vi "ma_SML RF Spectrum Units Conversion.vi"(6 "spectrum unit in":T2={"units"=enum."Adapt to spectral info", "peak scaling"=enum."rms", "psd?"=FALSE, "impedance(ohm)"=50.0} {"impedance(ohm)" format="%.2f"}, 8 "error in (no error)":errorcluster, 9 "unit conversion settings":T3={"units"=enum."dBV", "peak scaling"=enum."rms", "psd?"=FALSE, "impedance(ohm)"=50.0} {"impedance(ohm)" format="%.2f"}, 10 "spectral info in":T1 {"window" items=["Rectangle"=0, "Hanning"=1, "Hamming"=2, "Blackman-Harris"=3, "Exact Blackman"=4, "Blackman"=5, "Flat Top"=6, "4 Term B-Harris "=7, "7 Term B-Harris"=8, "Low Sidelobe"=9, "Blackman Nuttall"=11, "Triangle"=30, "Bartlett-Hanning"=31, "Bohman"=32, "Parzen"=33, "Welch"=34, "Kaiser"=60, "Dolph-Chebyshev"=61, "Gaussian"=62]}, 11 "power spectrum":T4={"f0"=0.0, "df"=1.0, "spectrum"=[]} {"spectrum" format="%.2f"; "df" format="%.2f"; "f0" format="%.2f"}) -> (0 "error out":errorcluster, 1 "units and label":cluster{"spectrum unit":string, "label":string}={"spectrum unit"="dBV", "label"="dBV rms^2"}, 2 "spectral info out":T1 {"window" items=["Rectangle"=0, "Hanning"=1, "Hamming"=2, "Blackman-Harris"=3, "Exact Blackman"=4, "Blackman"=5, "Flat Top"=6, "4 Term B-Harris "=7, "7 Term B-Harris"=8, "Low Sidelobe"=9, "Blackman Nuttall"=11, "Triangle"=30, "Bartlett-Hanning"=31, "Bohman"=32, "Parzen"=33, "Welch"=34, "Kaiser"=60, "Dolph-Chebyshev"=61, "Gaussian"=62]}, 3 "unit converted spectrum":T4={"f0"=0.0, "df"=1.0, "spectrum"=[]} {"spectrum" format="%.2f"; "df" format="%.2f"; "f0" format="%.2f"})   [LabVIEW 2020, in "NI_MAPro.lvlib"]
uses:
  NI_MAPro.lvlib
  ma_sml_Spectral Info.ctl
  ma_sml_Spectrum Cluster (real).ctl
panel:
  # "RF Spectrum Unit Conversion"
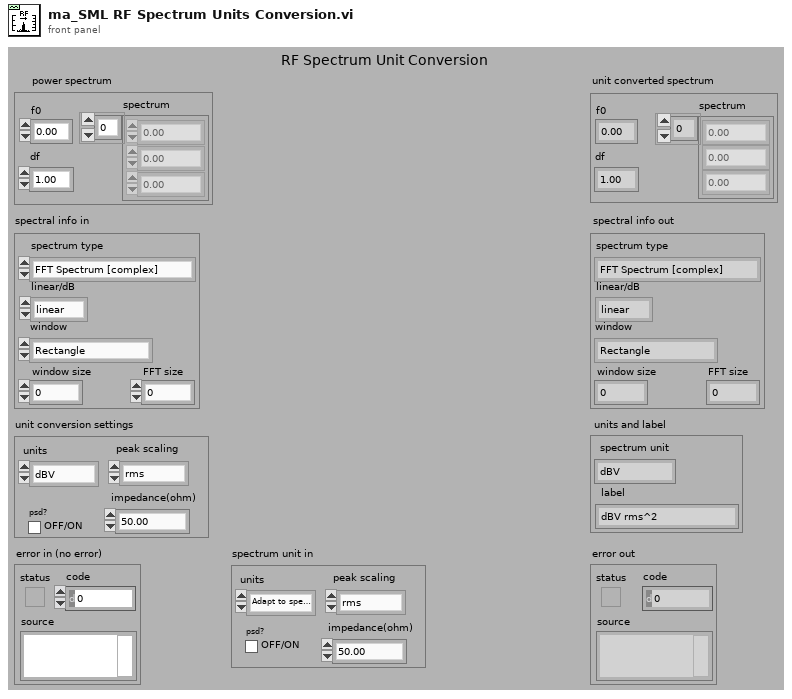
[diagram p1: front panel]
types:
  T1 = typedef "NI_MAPro.lvlib/ma_sml_Spectral Info.ctl" = cluster{"spectrum type":enum16{"FFT Spectrum [complex]", "Amplitude [Magnitude]", "Power [Magnitude^2]", "Cross Spectrum [complex]", "Frequency Response [Complex]"}, "linear/dB":enum16{"linear", "dB"}, "window":u16, "window size":i32, "FFT size":i32}
  T2 = cluster{"units":enum16{"V", "V^2", "W", "dBm", "dBW", "dBV", "dBmV", "dBuV", "Adapt to spectral info"}, "peak scaling":enum16{"rms", "pk"}, "psd?":bool, "impedance(ohm)":dbl}
  T3 = cluster{"units":enum16{"V", "V^2", "W", "dBm", "dBW", "dBV", "dBmV", "dBuV"}, "peak scaling":enum16{"rms", "pk"}, "psd?":bool, "impedance(ohm)":dbl}
  T4 = typedef "NI_MAPro.lvlib/ma_sml_Spectrum Cluster (real).ctl" = cluster{"f0":dbl, "df":dbl, "spectrum":dbl[]}
  T5 = enum16{"FFT Spectrum [complex]", "Amplitude [Magnitude]", "Power [Magnitude^2]", "Cross Spectrum [complex]", "Frequency Response [Complex]"}
  T6 = enum16{"V", "V^2", "W", "dBm", "dBW", "dBV", "dBmV", "dBuV"}
  T7 = enum16{"V", "V^2", "W", "dBm", "dBW", "dBV", "dBmV", "dBuV", "Adapt to spectral info"}
  T8 = enum16{"Linear To Sqr", "Sqr To Linear", "Linear To dB", "dB To Linear", "Sqr To dB", "dB To Sqr", "V^2 To W", "W To V^2", "dBV To dBW", "dBW To dBV", "dB To dBm", "dBm To dB", "dB To dBu", "dBu To dB"}[]
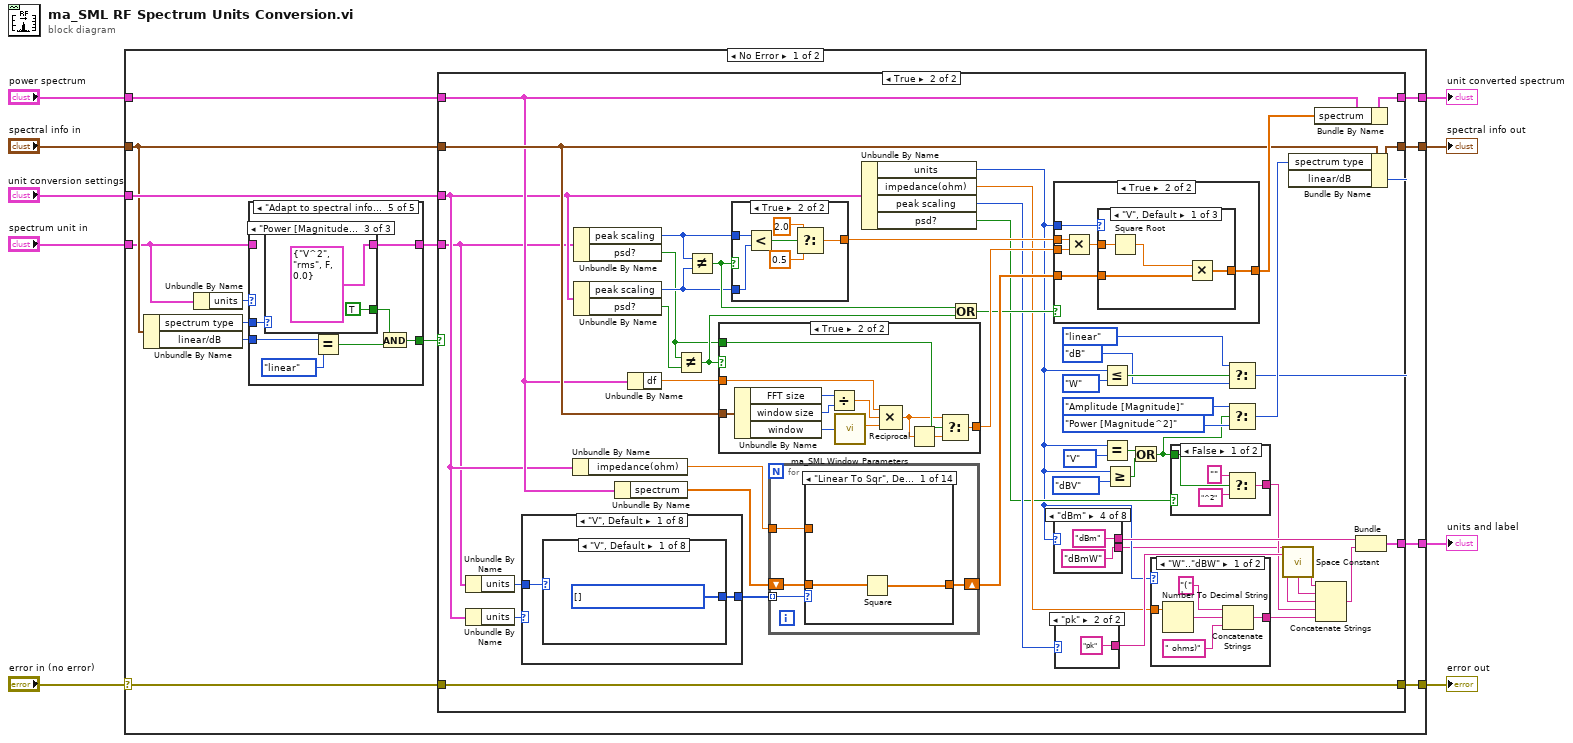
[diagram p0: block diagram]
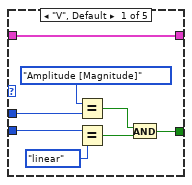
[diagram p2: hidden frame]
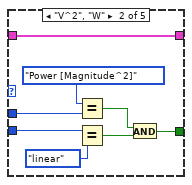
[diagram p3: hidden frame]
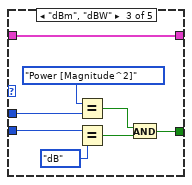
[diagram p4: hidden frame]
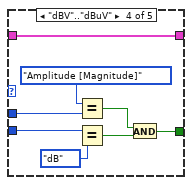
[diagram p5: hidden frame]
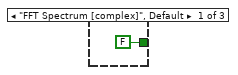
[diagram p6: hidden frame]
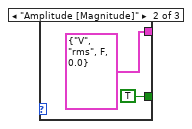
[diagram p7: hidden frame]
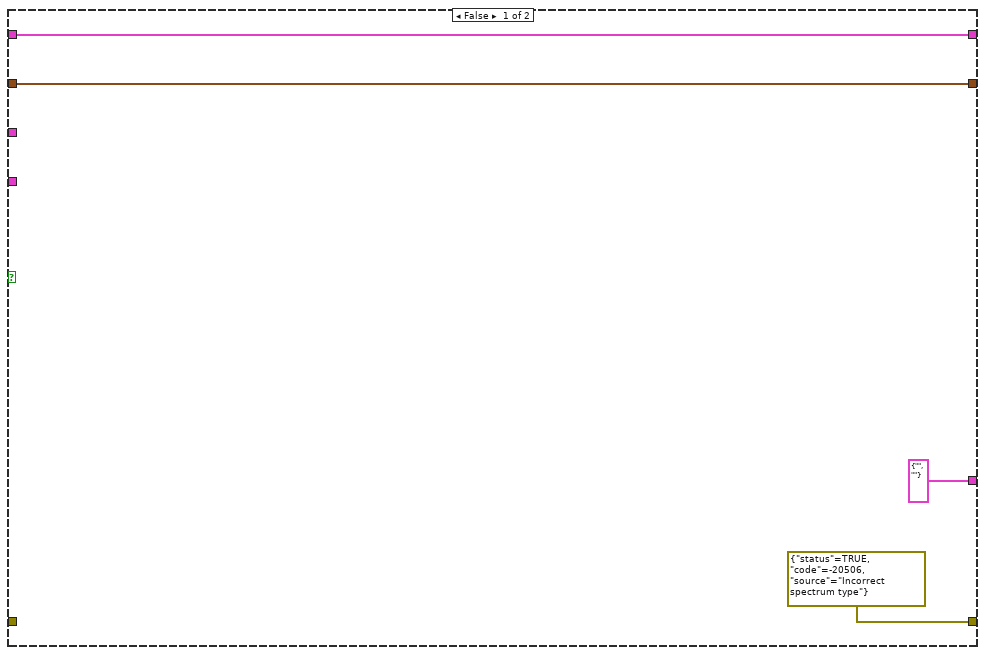
[diagram p8: hidden frame]
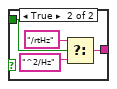
[diagram p9: hidden frame]
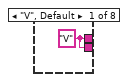
[diagram p10: hidden frame]
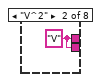
[diagram p11: hidden frame]
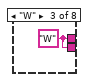
[diagram p12: hidden frame]
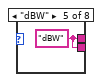
[diagram p13: hidden frame]
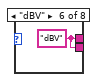
[diagram p14: hidden frame]
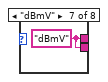
[diagram p15: hidden frame]
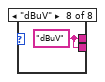
[diagram p16: hidden frame]
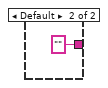
[diagram p17: hidden frame]
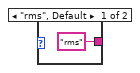
[diagram p18: hidden frame]
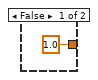
[diagram p19: hidden frame]
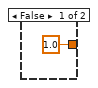
[diagram p20: hidden frame]
diagram:
  n1 = case shown="No Error" "error in (no error)" {
    selector: "error in (no error)" -> [w16 w322]
    tunnel: [w23 w320] -> w9
    tunnel: "power spectrum" -> [w22 w320]
    tunnel: "unit conversion settings" -> [w21 _]
    tunnel: "spectrum unit in" -> [w11 _]
    tunnel: [w20 cluster{string, string} {"", ""}] -> w5
    tunnel: "spectral info in" -> [w18 w321]
    tunnel: [w19 w321] -> w3
    tunnel: [w17 w322] -> w1
    frame No Error {
      n2 = Unbundle By Name(w18) -> ("spectrum type"=w14:T5, "linear/dB"=w13:enum16{"linear", "dB"})
      n3 = Unbundle By Name(w11) -> ("units"=w15:T7)
      n4 = case shown="\"Adapt to spectral info\"" w15 {
        tunnel: w14 -> [w26 w39 w42 w49 w62]
        tunnel: w13 -> [w25 w38 w41 w48 w60]
        tunnel: [w24 w34 w43 w50 w58] -> w12
        tunnel: w11 -> [w31 w35 w40 w55 _]
        tunnel: [w31 w35 w40 w55 w59] -> w10
        frame "V", Default {
          n5 = Equal?(x=T5."Amplitude [Magnitude]", y=w26) -> (x = y?=w27:bool)
          n6 = Equal?(x=w25, y=enum16{"linear", "dB"}."linear") -> (x = y?=w28:bool)
          n7 = And(x=w27, y=w28) -> (x .and. y?=w24:bool)
        }
        frame "V^2", "W" {
          n8 = Equal?(x=T5."Power [Magnitude^2]", y=w39) -> (x = y?=w32:bool)
          n9 = Equal?(x=w38, y=enum16{"linear", "dB"}."linear") -> (x = y?=w33:bool)
          n10 = And(x=w32, y=w33) -> (x .and. y?=w34:bool)
        }
        frame "dBm", "dBW" {
          n11 = Equal?(x=T5."Power [Magnitude^2]", y=w42) -> (x = y?=w44:bool)
          n12 = Equal?(x=w41, y=enum16{"linear", "dB"}."dB") -> (x = y?=w45:bool)
          n13 = And(x=w44, y=w45) -> (x .and. y?=w43:bool)
        }
        frame "dBV".."dBuV" {
          n14 = Equal?(x=T5."Amplitude [Magnitude]", y=w49) -> (x = y?=w51:bool)
          n15 = Equal?(x=w48, y=enum16{"linear", "dB"}."dB") -> (x = y?=w52:bool)
          n16 = And(x=w51, y=w52) -> (x .and. y?=w50:bool)
        }
        frame "Adapt to spectral info" {
          n17 = case shown="\"Power [Magnitude^2]\"" w62 {
            tunnel: [_ T2 {"units"=enum."V", "peak scaling"=enum."rms", "psd?"=FALSE, "impedance(ohm)"=0.0} ("spectrum unit in") T2 {"units"=enum."V^2", "peak scaling"=enum."rms", "psd?"=FALSE, "impedance(ohm)"=0.0} ("spectrum unit in")] -> w59
            tunnel: [FALSE TRUE TRUE] -> w56
            frame "FFT Spectrum [complex]", Default {
            }
            frame "Amplitude [Magnitude]" {
            }
            frame "Power [Magnitude^2]" {
            }
          }
          n18 = Equal?(x=w60, y=enum16{"linear", "dB"}."linear") -> (x = y?=w57:bool)
          n19 = And(x=w56, y=w57) -> (x .and. y?=w58:bool)
        }
      }
      n20 = case shown="True" w12 {
        tunnel: [w70 w120] -> w23
        tunnel: w22 -> [w70 w95]
        tunnel: w21 -> [_ w92]
        tunnel: w10 -> [_ w73]
        tunnel: [cluster{string, string} {"", ""} w101] -> w20
        tunnel: w18 -> [w69 w99]
        tunnel: [w69 w98] -> w19
        tunnel: [errorcluster {"status"=TRUE, "code"=-20506, "source"="Incorrect spectrum type"} ("Output Cluster") w97] -> w17
        tunnel: w16 -> [_ w97]
        frame False {
        }
        frame True {
          n21 = Unbundle By Name(w73) -> ("units"=w118:T7)
          n22 = Unbundle By Name(w92) -> ("units"=w119:T6)
          n23 = case shown="\"V\", Default" w119 {
            tunnel: w118 -> [w186 w195 w205 w215 w225 w235 w245 w255]
            tunnel: [w185 w196 w206 w216 w226 w236 w246 w256] -> w107
            frame "V", Default {
              n24 = case shown="\"V\", Default" w186 {
                tunnel: [w187 w188 w189 w190 w191 w192 w193 w194] -> w185
                frame "V", Default {
                  w187 = T8 [] items=["Linear To Sqr", "Sqr To Linear", "Linear To dB", "dB To Linear", "Sqr To dB", "dB To Sqr", "V^2 To W", "W To V^2", "dBV To dBW", "dBW To dBV", "dB To dBm", "dBm To dB", "dB To dBu", "dBu To dB"]
                }
                frame "V^2" {
                  w188 = T8 [enum."Sqr To Linear"] items=["Linear To Sqr", "Sqr To Linear", "Linear To dB", "dB To Linear", "Sqr To dB", "dB To Sqr", "V^2 To W", "W To V^2", "dBV To dBW", "dBW To dBV", "dB To dBm", "dBm To dB", "dB To dBu", "dBu To dB"]
                }
                frame "W" {
                  w189 = T8 [enum."W To V^2", enum."Sqr To Linear"] items=["Linear To Sqr", "Sqr To Linear", "Linear To dB", "dB To Linear", "Sqr To dB", "dB To Sqr", "V^2 To W", "W To V^2", "dBV To dBW", "dBW To dBV", "dB To dBm", "dBm To dB", "dB To dBu", "dBu To dB"]
                }
                frame "dBm" {
                  w190 = T8 [enum."dBm To dB", enum."dBW To dBV", enum."dB To Linear"] items=["Linear To Sqr", "Sqr To Linear", "Linear To dB", "dB To Linear", "Sqr To dB", "dB To Sqr", "V^2 To W", "W To V^2", "dBV To dBW", "dBW To dBV", "dB To dBm", "dBm To dB", "dB To dBu", "dBu To dB"]
                }
                frame "dBW" {
                  w191 = T8 [enum."dBW To dBV", enum."dB To Linear"] items=["Linear To Sqr", "Sqr To Linear", "Linear To dB", "dB To Linear", "Sqr To dB", "dB To Sqr", "V^2 To W", "W To V^2", "dBV To dBW", "dBW To dBV", "dB To dBm", "dBm To dB", "dB To dBu", "dBu To dB"]
                }
                frame "dBV" {
                  w192 = T8 [enum."dB To Linear"] items=["Linear To Sqr", "Sqr To Linear", "Linear To dB", "dB To Linear", "Sqr To dB", "dB To Sqr", "V^2 To W", "W To V^2", "dBV To dBW", "dBW To dBV", "dB To dBm", "dBm To dB", "dB To dBu", "dBu To dB"]
                }
                frame "dBmV" {
                  w193 = T8 [enum."dBu To dB", enum."dB To Linear"] items=["Linear To Sqr", "Sqr To Linear", "Linear To dB", "dB To Linear", "Sqr To dB", "dB To Sqr", "V^2 To W", "W To V^2", "dBV To dBW", "dBW To dBV", "dB To dBm", "dBm To dB", "dB To dBu", "dBu To dB"]
                }
                frame "dBuV" {
                  w194 = T8 [enum."dBu To dB", enum."dBu To dB", enum."dB To Linear"] items=["Linear To Sqr", "Sqr To Linear", "Linear To dB", "dB To Linear", "Sqr To dB", "dB To Sqr", "V^2 To W", "W To V^2", "dBV To dBW", "dBW To dBV", "dB To dBm", "dBm To dB", "dB To dBu", "dBu To dB"]
                }
              }
            }
            frame "V^2" {
              n25 = case shown="\"V\", Default" w195 {
                tunnel: [w197 w198 w199 w200 w201 w202 w203 w204] -> w196
                frame "V", Default {
                  w197 = T8 [enum."Linear To Sqr"] items=["Linear To Sqr", "Sqr To Linear", "Linear To dB", "dB To Linear", "Sqr To dB", "dB To Sqr", "V^2 To W", "W To V^2", "dBV To dBW", "dBW To dBV", "dB To dBm", "dBm To dB", "dB To dBu", "dBu To dB"]
                }
                frame "V^2" {
                  w198 = T8 [] items=["Linear To Sqr", "Sqr To Linear", "Linear To dB", "dB To Linear", "Sqr To dB", "dB To Sqr", "V^2 To W", "W To V^2", "dBV To dBW", "dBW To dBV", "dB To dBm", "dBm To dB", "dB To dBu", "dBu To dB"]
                }
                frame "W" {
                  w199 = T8 [enum."W To V^2"] items=["Linear To Sqr", "Sqr To Linear", "Linear To dB", "dB To Linear", "Sqr To dB", "dB To Sqr", "V^2 To W", "W To V^2", "dBV To dBW", "dBW To dBV", "dB To dBm", "dBm To dB", "dB To dBu", "dBu To dB"]
                }
                frame "dBm" {
                  w200 = T8 [enum."dBm To dB", enum."dBW To dBV", enum."dB To Sqr"] items=["Linear To Sqr", "Sqr To Linear", "Linear To dB", "dB To Linear", "Sqr To dB", "dB To Sqr", "V^2 To W", "W To V^2", "dBV To dBW", "dBW To dBV", "dB To dBm", "dBm To dB", "dB To dBu", "dBu To dB"]
                }
                frame "dBW" {
                  w201 = T8 [enum."dBW To dBV", enum."dB To Sqr"] items=["Linear To Sqr", "Sqr To Linear", "Linear To dB", "dB To Linear", "Sqr To dB", "dB To Sqr", "V^2 To W", "W To V^2", "dBV To dBW", "dBW To dBV", "dB To dBm", "dBm To dB", "dB To dBu", "dBu To dB"]
                }
                frame "dBV" {
                  w202 = T8 [enum."dB To Sqr"] items=["Linear To Sqr", "Sqr To Linear", "Linear To dB", "dB To Linear", "Sqr To dB", "dB To Sqr", "V^2 To W", "W To V^2", "dBV To dBW", "dBW To dBV", "dB To dBm", "dBm To dB", "dB To dBu", "dBu To dB"]
                }
                frame "dBmV" {
                  w203 = T8 [enum."dBu To dB", enum."dB To Sqr"] items=["Linear To Sqr", "Sqr To Linear", "Linear To dB", "dB To Linear", "Sqr To dB", "dB To Sqr", "V^2 To W", "W To V^2", "dBV To dBW", "dBW To dBV", "dB To dBm", "dBm To dB", "dB To dBu", "dBu To dB"]
                }
                frame "dBuV" {
                  w204 = T8 [enum."dBu To dB", enum."dBu To dB", enum."dB To Sqr"] items=["Linear To Sqr", "Sqr To Linear", "Linear To dB", "dB To Linear", "Sqr To dB", "dB To Sqr", "V^2 To W", "W To V^2", "dBV To dBW", "dBW To dBV", "dB To dBm", "dBm To dB", "dB To dBu", "dBu To dB"]
                }
              }
            }
            frame "W" {
              n26 = case shown="\"V\", Default" w205 {
                tunnel: [w207 w208 w209 w210 w211 w212 w213 w214] -> w206
                frame "V", Default {
                  w207 = T8 [enum."Linear To Sqr", enum."V^2 To W"] items=["Linear To Sqr", "Sqr To Linear", "Linear To dB", "dB To Linear", "Sqr To dB", "dB To Sqr", "V^2 To W", "W To V^2", "dBV To dBW", "dBW To dBV", "dB To dBm", "dBm To dB", "dB To dBu", "dBu To dB"]
                }
                frame "V^2" {
                  w208 = T8 [enum."V^2 To W"] items=["Linear To Sqr", "Sqr To Linear", "Linear To dB", "dB To Linear", "Sqr To dB", "dB To Sqr", "V^2 To W", "W To V^2", "dBV To dBW", "dBW To dBV", "dB To dBm", "dBm To dB", "dB To dBu", "dBu To dB"]
                }
                frame "W" {
                  w209 = T8 [] items=["Linear To Sqr", "Sqr To Linear", "Linear To dB", "dB To Linear", "Sqr To dB", "dB To Sqr", "V^2 To W", "W To V^2", "dBV To dBW", "dBW To dBV", "dB To dBm", "dBm To dB", "dB To dBu", "dBu To dB"]
                }
                frame "dBm" {
                  w210 = T8 [enum."dBm To dB", enum."dB To Sqr"] items=["Linear To Sqr", "Sqr To Linear", "Linear To dB", "dB To Linear", "Sqr To dB", "dB To Sqr", "V^2 To W", "W To V^2", "dBV To dBW", "dBW To dBV", "dB To dBm", "dBm To dB", "dB To dBu", "dBu To dB"]
                }
                frame "dBW" {
                  w211 = T8 [enum."dB To Sqr"] items=["Linear To Sqr", "Sqr To Linear", "Linear To dB", "dB To Linear", "Sqr To dB", "dB To Sqr", "V^2 To W", "W To V^2", "dBV To dBW", "dBW To dBV", "dB To dBm", "dBm To dB", "dB To dBu", "dBu To dB"]
                }
                frame "dBV" {
                  w212 = T8 [enum."dBV To dBW", enum."dB To Sqr"] items=["Linear To Sqr", "Sqr To Linear", "Linear To dB", "dB To Linear", "Sqr To dB", "dB To Sqr", "V^2 To W", "W To V^2", "dBV To dBW", "dBW To dBV", "dB To dBm", "dBm To dB", "dB To dBu", "dBu To dB"]
                }
                frame "dBmV" {
                  w213 = T8 [enum."dBu To dB", enum."dBV To dBW", enum."dB To Sqr"] items=["Linear To Sqr", "Sqr To Linear", "Linear To dB", "dB To Linear", "Sqr To dB", "dB To Sqr", "V^2 To W", "W To V^2", "dBV To dBW", "dBW To dBV", "dB To dBm", "dBm To dB", "dB To dBu", "dBu To dB"]
                }
                frame "dBuV" {
                  w214 = T8 [enum."dBu To dB", enum."dBu To dB", enum."dBV To dBW", enum."dB To Sqr"] items=["Linear To Sqr", "Sqr To Linear", "Linear To dB", "dB To Linear", "Sqr To dB", "dB To Sqr", "V^2 To W", "W To V^2", "dBV To dBW", "dBW To dBV", "dB To dBm", "dBm To dB", "dB To dBu", "dBu To dB"]
                }
              }
            }
            frame "dBm" {
              n27 = case shown="\"V\", Default" w215 {
                tunnel: [w217 w218 w219 w220 w221 w222 w223 w224] -> w216
                frame "V", Default {
                  w217 = T8 [enum."Linear To dB", enum."dBV To dBW", enum."dB To dBm"] items=["Linear To Sqr", "Sqr To Linear", "Linear To dB", "dB To Linear", "Sqr To dB", "dB To Sqr", "V^2 To W", "W To V^2", "dBV To dBW", "dBW To dBV", "dB To dBm", "dBm To dB", "dB To dBu", "dBu To dB"]
                }
                frame "V^2" {
                  w218 = T8 [enum."Sqr To dB", enum."dBV To dBW", enum."dB To dBm"] items=["Linear To Sqr", "Sqr To Linear", "Linear To dB", "dB To Linear", "Sqr To dB", "dB To Sqr", "V^2 To W", "W To V^2", "dBV To dBW", "dBW To dBV", "dB To dBm", "dBm To dB", "dB To dBu", "dBu To dB"]
                }
                frame "W" {
                  w219 = T8 [enum."Sqr To dB", enum."dB To dBm"] items=["Linear To Sqr", "Sqr To Linear", "Linear To dB", "dB To Linear", "Sqr To dB", "dB To Sqr", "V^2 To W", "W To V^2", "dBV To dBW", "dBW To dBV", "dB To dBm", "dBm To dB", "dB To dBu", "dBu To dB"]
                }
                frame "dBm" {
                  w220 = T8 [] items=["Linear To Sqr", "Sqr To Linear", "Linear To dB", "dB To Linear", "Sqr To dB", "dB To Sqr", "V^2 To W", "W To V^2", "dBV To dBW", "dBW To dBV", "dB To dBm", "dBm To dB", "dB To dBu", "dBu To dB"]
                }
                frame "dBW" {
                  w221 = T8 [enum."dB To dBm"] items=["Linear To Sqr", "Sqr To Linear", "Linear To dB", "dB To Linear", "Sqr To dB", "dB To Sqr", "V^2 To W", "W To V^2", "dBV To dBW", "dBW To dBV", "dB To dBm", "dBm To dB", "dB To dBu", "dBu To dB"]
                }
                frame "dBV" {
                  w222 = T8 [enum."dBV To dBW", enum."dB To dBm"] items=["Linear To Sqr", "Sqr To Linear", "Linear To dB", "dB To Linear", "Sqr To dB", "dB To Sqr", "V^2 To W", "W To V^2", "dBV To dBW", "dBW To dBV", "dB To dBm", "dBm To dB", "dB To dBu", "dBu To dB"]
                }
                frame "dBmV" {
                  w223 = T8 [enum."dBV To dBW", enum."dBm To dB"] items=["Linear To Sqr", "Sqr To Linear", "Linear To dB", "dB To Linear", "Sqr To dB", "dB To Sqr", "V^2 To W", "W To V^2", "dBV To dBW", "dBW To dBV", "dB To dBm", "dBm To dB", "dB To dBu", "dBu To dB"]
                }
                frame "dBuV" {
                  w224 = T8 [enum."dBV To dBW", enum."dBm To dB", enum."dBu To dB"] items=["Linear To Sqr", "Sqr To Linear", "Linear To dB", "dB To Linear", "Sqr To dB", "dB To Sqr", "V^2 To W", "W To V^2", "dBV To dBW", "dBW To dBV", "dB To dBm", "dBm To dB", "dB To dBu", "dBu To dB"]
                }
              }
            }
            frame "dBW" {
              n28 = case shown="\"V\", Default" w225 {
                tunnel: [w227 w228 w229 w230 w231 w232 w233 w234] -> w226
                frame "V", Default {
                  w227 = T8 [enum."Linear To dB", enum."dBV To dBW"] items=["Linear To Sqr", "Sqr To Linear", "Linear To dB", "dB To Linear", "Sqr To dB", "dB To Sqr", "V^2 To W", "W To V^2", "dBV To dBW", "dBW To dBV", "dB To dBm", "dBm To dB", "dB To dBu", "dBu To dB"]
                }
                frame "V^2" {
                  w228 = T8 [enum."Sqr To dB", enum."dBV To dBW"] items=["Linear To Sqr", "Sqr To Linear", "Linear To dB", "dB To Linear", "Sqr To dB", "dB To Sqr", "V^2 To W", "W To V^2", "dBV To dBW", "dBW To dBV", "dB To dBm", "dBm To dB", "dB To dBu", "dBu To dB"]
                }
                frame "W" {
                  w229 = T8 [enum."Sqr To dB"] items=["Linear To Sqr", "Sqr To Linear", "Linear To dB", "dB To Linear", "Sqr To dB", "dB To Sqr", "V^2 To W", "W To V^2", "dBV To dBW", "dBW To dBV", "dB To dBm", "dBm To dB", "dB To dBu", "dBu To dB"]
                }
                frame "dBm" {
                  w230 = T8 [enum."dBm To dB"] items=["Linear To Sqr", "Sqr To Linear", "Linear To dB", "dB To Linear", "Sqr To dB", "dB To Sqr", "V^2 To W", "W To V^2", "dBV To dBW", "dBW To dBV", "dB To dBm", "dBm To dB", "dB To dBu", "dBu To dB"]
                }
                frame "dBW" {
                  w231 = T8 [] items=["Linear To Sqr", "Sqr To Linear", "Linear To dB", "dB To Linear", "Sqr To dB", "dB To Sqr", "V^2 To W", "W To V^2", "dBV To dBW", "dBW To dBV", "dB To dBm", "dBm To dB", "dB To dBu", "dBu To dB"]
                }
                frame "dBV" {
                  w232 = T8 [enum."dBV To dBW"] items=["Linear To Sqr", "Sqr To Linear", "Linear To dB", "dB To Linear", "Sqr To dB", "dB To Sqr", "V^2 To W", "W To V^2", "dBV To dBW", "dBW To dBV", "dB To dBm", "dBm To dB", "dB To dBu", "dBu To dB"]
                }
                frame "dBmV" {
                  w233 = T8 [enum."dBV To dBW", enum."dBu To dB"] items=["Linear To Sqr", "Sqr To Linear", "Linear To dB", "dB To Linear", "Sqr To dB", "dB To Sqr", "V^2 To W", "W To V^2", "dBV To dBW", "dBW To dBV", "dB To dBm", "dBm To dB", "dB To dBu", "dBu To dB"]
                }
                frame "dBuV" {
                  w234 = T8 [enum."dBV To dBW", enum."dBu To dB", enum."dBu To dB"] items=["Linear To Sqr", "Sqr To Linear", "Linear To dB", "dB To Linear", "Sqr To dB", "dB To Sqr", "V^2 To W", "W To V^2", "dBV To dBW", "dBW To dBV", "dB To dBm", "dBm To dB", "dB To dBu", "dBu To dB"]
                }
              }
            }
            frame "dBV" {
              n29 = case shown="\"V\", Default" w235 {
                tunnel: [w237 w238 w239 w240 w241 w242 w243 w244] -> w236
                frame "V", Default {
                  w237 = T8 [enum."Linear To dB"] items=["Linear To Sqr", "Sqr To Linear", "Linear To dB", "dB To Linear", "Sqr To dB", "dB To Sqr", "V^2 To W", "W To V^2", "dBV To dBW", "dBW To dBV", "dB To dBm", "dBm To dB", "dB To dBu", "dBu To dB"]
                }
                frame "V^2" {
                  w238 = T8 [enum."Sqr To dB"] items=["Linear To Sqr", "Sqr To Linear", "Linear To dB", "dB To Linear", "Sqr To dB", "dB To Sqr", "V^2 To W", "W To V^2", "dBV To dBW", "dBW To dBV", "dB To dBm", "dBm To dB", "dB To dBu", "dBu To dB"]
                }
                frame "W" {
                  w239 = T8 [enum."Sqr To dB", enum."dBW To dBV"] items=["Linear To Sqr", "Sqr To Linear", "Linear To dB", "dB To Linear", "Sqr To dB", "dB To Sqr", "V^2 To W", "W To V^2", "dBV To dBW", "dBW To dBV", "dB To dBm", "dBm To dB", "dB To dBu", "dBu To dB"]
                }
                frame "dBm" {
                  w240 = T8 [enum."dBW To dBV", enum."dBm To dB"] items=["Linear To Sqr", "Sqr To Linear", "Linear To dB", "dB To Linear", "Sqr To dB", "dB To Sqr", "V^2 To W", "W To V^2", "dBV To dBW", "dBW To dBV", "dB To dBm", "dBm To dB", "dB To dBu", "dBu To dB"]
                }
                frame "dBW" {
                  w241 = T8 [enum."dBW To dBV"] items=["Linear To Sqr", "Sqr To Linear", "Linear To dB", "dB To Linear", "Sqr To dB", "dB To Sqr", "V^2 To W", "W To V^2", "dBV To dBW", "dBW To dBV", "dB To dBm", "dBm To dB", "dB To dBu", "dBu To dB"]
                }
                frame "dBV" {
                  w242 = T8 [] items=["Linear To Sqr", "Sqr To Linear", "Linear To dB", "dB To Linear", "Sqr To dB", "dB To Sqr", "V^2 To W", "W To V^2", "dBV To dBW", "dBW To dBV", "dB To dBm", "dBm To dB", "dB To dBu", "dBu To dB"]
                }
                frame "dBmV" {
                  w243 = T8 [enum."dBu To dB"] items=["Linear To Sqr", "Sqr To Linear", "Linear To dB", "dB To Linear", "Sqr To dB", "dB To Sqr", "V^2 To W", "W To V^2", "dBV To dBW", "dBW To dBV", "dB To dBm", "dBm To dB", "dB To dBu", "dBu To dB"]
                }
                frame "dBuV" {
                  w244 = T8 [enum."dBu To dB", enum."dBu To dB"] items=["Linear To Sqr", "Sqr To Linear", "Linear To dB", "dB To Linear", "Sqr To dB", "dB To Sqr", "V^2 To W", "W To V^2", "dBV To dBW", "dBW To dBV", "dB To dBm", "dBm To dB", "dB To dBu", "dBu To dB"]
                }
              }
            }
            frame "dBmV" {
              n30 = case shown="\"V\", Default" w245 {
                tunnel: [w247 w248 w249 w250 w251 w252 w253 w254] -> w246
                frame "V", Default {
                  w247 = T8 [enum."Linear To dB", enum."dB To dBu"] items=["Linear To Sqr", "Sqr To Linear", "Linear To dB", "dB To Linear", "Sqr To dB", "dB To Sqr", "V^2 To W", "W To V^2", "dBV To dBW", "dBW To dBV", "dB To dBm", "dBm To dB", "dB To dBu", "dBu To dB"]
                }
                frame "V^2" {
                  w248 = T8 [enum."Sqr To dB", enum."dB To dBu"] items=["Linear To Sqr", "Sqr To Linear", "Linear To dB", "dB To Linear", "Sqr To dB", "dB To Sqr", "V^2 To W", "W To V^2", "dBV To dBW", "dBW To dBV", "dB To dBm", "dBm To dB", "dB To dBu", "dBu To dB"]
                }
                frame "W" {
                  w249 = T8 [enum."Sqr To dB", enum."dBW To dBV", enum."dB To dBu"] items=["Linear To Sqr", "Sqr To Linear", "Linear To dB", "dB To Linear", "Sqr To dB", "dB To Sqr", "V^2 To W", "W To V^2", "dBV To dBW", "dBW To dBV", "dB To dBm", "dBm To dB", "dB To dBu", "dBu To dB"]
                }
                frame "dBm" {
                  w250 = T8 [enum."dBW To dBV", enum."dB To dBm"] items=["Linear To Sqr", "Sqr To Linear", "Linear To dB", "dB To Linear", "Sqr To dB", "dB To Sqr", "V^2 To W", "W To V^2", "dBV To dBW", "dBW To dBV", "dB To dBm", "dBm To dB", "dB To dBu", "dBu To dB"]
                }
                frame "dBW" {
                  w251 = T8 [enum."dBW To dBV", enum."dB To dBu"] items=["Linear To Sqr", "Sqr To Linear", "Linear To dB", "dB To Linear", "Sqr To dB", "dB To Sqr", "V^2 To W", "W To V^2", "dBV To dBW", "dBW To dBV", "dB To dBm", "dBm To dB", "dB To dBu", "dBu To dB"]
                }
                frame "dBV" {
                  w252 = T8 [enum."dB To dBu"] items=["Linear To Sqr", "Sqr To Linear", "Linear To dB", "dB To Linear", "Sqr To dB", "dB To Sqr", "V^2 To W", "W To V^2", "dBV To dBW", "dBW To dBV", "dB To dBm", "dBm To dB", "dB To dBu", "dBu To dB"]
                }
                frame "dBmV" {
                  w253 = T8 [] items=["Linear To Sqr", "Sqr To Linear", "Linear To dB", "dB To Linear", "Sqr To dB", "dB To Sqr", "V^2 To W", "W To V^2", "dBV To dBW", "dBW To dBV", "dB To dBm", "dBm To dB", "dB To dBu", "dBu To dB"]
                }
                frame "dBuV" {
                  w254 = T8 [enum."dBu To dB"] items=["Linear To Sqr", "Sqr To Linear", "Linear To dB", "dB To Linear", "Sqr To dB", "dB To Sqr", "V^2 To W", "W To V^2", "dBV To dBW", "dBW To dBV", "dB To dBm", "dBm To dB", "dB To dBu", "dBu To dB"]
                }
              }
            }
            frame "dBuV" {
              n31 = case shown="\"V\", Default" w255 {
                tunnel: [w257 w258 w259 w260 w261 w262 w263 w264] -> w256
                frame "V", Default {
                  w257 = T8 [enum."Linear To dB", enum."dB To dBu", enum."dB To dBu"] items=["Linear To Sqr", "Sqr To Linear", "Linear To dB", "dB To Linear", "Sqr To dB", "dB To Sqr", "V^2 To W", "W To V^2", "dBV To dBW", "dBW To dBV", "dB To dBm", "dBm To dB", "dB To dBu", "dBu To dB"]
                }
                frame "V^2" {
                  w258 = T8 [enum."Sqr To dB", enum."dB To dBu", enum."dB To dBu"] items=["Linear To Sqr", "Sqr To Linear", "Linear To dB", "dB To Linear", "Sqr To dB", "dB To Sqr", "V^2 To W", "W To V^2", "dBV To dBW", "dBW To dBV", "dB To dBm", "dBm To dB", "dB To dBu", "dBu To dB"]
                }
                frame "W" {
                  w259 = T8 [enum."Sqr To dB", enum."dBW To dBV", enum."dB To dBu", enum."dB To dBu"] items=["Linear To Sqr", "Sqr To Linear", "Linear To dB", "dB To Linear", "Sqr To dB", "dB To Sqr", "V^2 To W", "W To V^2", "dBV To dBW", "dBW To dBV", "dB To dBm", "dBm To dB", "dB To dBu", "dBu To dB"]
                }
                frame "dBm" {
                  w260 = T8 [enum."dBW To dBV", enum."dB To dBm", enum."dB To dBu"] items=["Linear To Sqr", "Sqr To Linear", "Linear To dB", "dB To Linear", "Sqr To dB", "dB To Sqr", "V^2 To W", "W To V^2", "dBV To dBW", "dBW To dBV", "dB To dBm", "dBm To dB", "dB To dBu", "dBu To dB"]
                }
                frame "dBW" {
                  w261 = T8 [enum."dBW To dBV", enum."dB To dBu", enum."dB To dBu"] items=["Linear To Sqr", "Sqr To Linear", "Linear To dB", "dB To Linear", "Sqr To dB", "dB To Sqr", "V^2 To W", "W To V^2", "dBV To dBW", "dBW To dBV", "dB To dBm", "dBm To dB", "dB To dBu", "dBu To dB"]
                }
                frame "dBV" {
                  w262 = T8 [enum."dB To dBu", enum."dB To dBu"] items=["Linear To Sqr", "Sqr To Linear", "Linear To dB", "dB To Linear", "Sqr To dB", "dB To Sqr", "V^2 To W", "W To V^2", "dBV To dBW", "dBW To dBV", "dB To dBm", "dBm To dB", "dB To dBu", "dBu To dB"]
                }
                frame "dBmV" {
                  w263 = T8 [enum."dB To dBu"] items=["Linear To Sqr", "Sqr To Linear", "Linear To dB", "dB To Linear", "Sqr To dB", "dB To Sqr", "V^2 To W", "W To V^2", "dBV To dBW", "dBW To dBV", "dB To dBm", "dBm To dB", "dB To dBu", "dBu To dB"]
                }
                frame "dBuV" {
                  w264 = T8 [] items=["Linear To Sqr", "Sqr To Linear", "Linear To dB", "dB To Linear", "Sqr To dB", "dB To Sqr", "V^2 To W", "W To V^2", "dBV To dBW", "dBW To dBV", "dB To dBm", "dBm To dB", "dB To dBu", "dBu To dB"]
                }
              }
            }
          }
          n32 = Unbundle By Name(w92) -> ("impedance(ohm)"=w93:dbl)
          n33 = Unbundle By Name(w73) -> ("peak scaling"=w111:enum16{"rms", "pk"}, "psd?"=w96:bool)
          n34 = Unbundle By Name(w92) -> ("peak scaling"=w110:enum16{"rms", "pk"}, "psd?"=w109:bool)
          n35 = Unbundle By Name(w95) -> ("spectrum"=w108:dbl[])
          n36 = Unbundle By Name(w95) -> ("df"=w94:dbl)
          n37 = Not Equal?(x=w96, y=w109) -> (x != y?=w115:bool)
          n38 = Not Equal?(x=w111, y=w110) -> (x != y?=w116:bool)
          n39 = case shown="True" w115 {
            tunnel: w96 -> [_ w151]
            tunnel: w99 -> [_ w157]
            tunnel: [1.0 w150] -> w113
            tunnel: w94 -> [_ w149]
            frame False {
            }
            frame True {
              n40 = Unbundle By Name(w157) -> ("FFT size"=w156:i32, "window size"=w155:i32, "window"=w154:u16)
              n41 = Divide(x=w156, y=w155) -> (x/y=w153:dbl)
              n42 = call "ma_SML Window Parameters.vi"("window"=w154) -> ("ENBW"=w152:dbl)  [unwired: 3 out]
              n43 = Compound Arithmetic op=MULTIPLY(w149, w153, w152) -> (w147:dbl)
              n44 = Reciprocal(x=w147) -> (1/x=w148:dbl)
              n45 = Select(t=w147, s=w151, f=w148) -> (s? t:f=w150:dbl)
            }
          }
          n46 = case shown="True" w116 {
            tunnel: w111 -> [_ w161]
            tunnel: w110 -> [_ w160]
            tunnel: [1.0 w159] -> w114
            frame False {
            }
            frame True {
              n47 = Less?(x=w161, y=w160) -> (x < y?=w163:bool)
              n48 = Select(t=2.0, s=w163, f=0.5) -> (s? t:f=w159:dbl)
            }
          }
          n49 = for {
            shift-right: [w267] -> w117
            shift-left: w108 -> [w268]
            tunnel: w93 -> [w266]
            tunnel: w107 -> [w265] mode=indexing
            n50 = case shown="\"Linear To Sqr\", Default" w265 {
              tunnel: w268 -> [w270 w272 w276 w278 w284 w287 w291 w293 w296 w304 w308 w312 w315 w318]
              tunnel: [w269 w271 w275 w277 w283 w286 w290 w294 w299 w302 w309 w311 w314 w316] -> w267
              tunnel: w266 -> [_ _ _ _ _ _ w289 w292 w295 w301 _ _ _ _]
              frame "Linear To Sqr", Default {
                n51 = Square(x=w270) -> (x^2=w269:dbl[])
              }
              frame "Sqr To Linear" {
                n52 = Square Root(x=w272) -> (sqrt(x)=w271:dbl[])
              }
              frame "Linear To dB" {
                n53 = Logarithm Base 10(1:w276) -> (0:w274:dbl[])
                n54 = Multiply(x=20.0, y=w274) -> (x*y=w275:dbl[])
              }
              frame "dB To Linear" {
                n55 = Divide(x=w278, y=20.0) -> (x/y=w279:dbl[])
                n56 = Power Of 10(x=w279) -> (10^x=w277:dbl[])
              }
              frame "Sqr To dB" {
                n57 = Logarithm Base 10(1:w284) -> (0:w282:dbl[])
                n58 = Multiply(x=10.0, y=w282) -> (x*y=w283:dbl[])
              }
              frame "dB To Sqr" {
                n59 = Divide(x=w287, y=10.0) -> (x/y=w285:dbl[])
                n60 = Power Of 10(x=w285) -> (10^x=w286:dbl[])
              }
              frame "V^2 To W" {
                n61 = Divide(x=w291, y=w289) -> (x/y=w290:dbl[])
              }
              frame "W To V^2" {
                n62 = Multiply(x=w292, y=w293) -> (x*y=w294:dbl[])
              }
              frame "dBV To dBW" {
                n63 = Logarithm Base 10(1:w295) -> (0:w298:dbl)
                n64 = Multiply(x=10.0 ("y"), y=w298) -> (x*y=w300:dbl)
                n65 = Subtract(x=w296, y=w300) -> (x-y=w299:dbl[])
              }
              frame "dBW To dBV" {
                n66 = Logarithm Base 10(1:w301) -> (0:w306:dbl)
                n67 = Multiply(x=10.0 ("y"), y=w306) -> (x*y=w303:dbl)
                n68 = Add(x=w303, y=w304) -> (x+y=w302:dbl[])
              }
              frame "dB To dBm" {
                n69 = Add(x=w308, y=30.0) -> (x+y=w309:dbl[])
              }
              frame "dBm To dB" {
                n70 = Subtract(x=w312, y=30.0) -> (x-y=w311:dbl[])
              }
              frame "dB To dBu" {
                n71 = Add(x=w315, y=60.0) -> (x+y=w314:dbl[])
              }
              frame "dBu To dB" {
                n72 = Subtract(x=w318, y=60.0) -> (x-y=w316:dbl[])
              }
            }
          }
          n73 = Unbundle By Name(w92) -> ("units"=w76:T6, "impedance(ohm)"=w105:dbl, "peak scaling"=w90:enum16{"rms", "pk"}, "psd?"=w80:bool)
          n74 = Or(x=w116, y=w115) -> (x .or. y?=w112:bool)
          n75 = case shown="True" w112 {
            tunnel: w117 -> [w165 w171]
            tunnel: [w165 w170] -> w100
            tunnel: w114 -> [_ w167]
            tunnel: w113 -> [_ w169]
            tunnel: w76 -> [_ w166]
            frame False {
            }
            frame True {
              n76 = Multiply(x=w167, y=w169) -> (x*y=w168:dbl)
              n77 = case shown="\"V\", Default" w166 {
                tunnel: w168 -> [w175 w177 w181]
                tunnel: w171 -> [w173 w178 w184]
                tunnel: [w172 w176 w183] -> w170
                frame "V", Default {
                  n78 = Square Root(x=w175) -> (sqrt(x)=w174:dbl)
                  n79 = Multiply(x=w174, y=w173) -> (x*y=w172:dbl[])
                }
                frame "V^2", "W" {
                  n80 = Multiply(x=w177, y=w178) -> (x*y=w176:dbl[])
                }
                frame "dBm".."dBuV" {
                  n81 = Logarithm Base 10(1:w181) -> (0:w182:dbl)
                  n82 = Multiply(x=w182, y=10.0) -> (x*y=w180:dbl)
                  n83 = Add(x=w180, y=w184) -> (x+y=w183:dbl[])
                }
              }
            }
          }
          n84 = case shown="\"dBm\"" w76 {
            tunnel: [w129 w130 w131 "dBm" w134 w135 w136 w137] -> w103
            tunnel: [w129 w130 w131 "dBmW" w134 w135 w136 w137] -> w72
            frame "V", Default {
              w129 = "V"
            }
            frame "V^2" {
              w130 = "V"
            }
            frame "W" {
              w131 = "W"
            }
            frame "dBm" {
            }
            frame "dBW" {
              w134 = "dBW"
            }
            frame "dBV" {
              w135 = "dBV"
            }
            frame "dBmV" {
              w136 = "dBmV"
            }
            frame "dBuV" {
              w137 = "dBuV"
            }
          }
          n85 = case shown="\"pk\"" w90 {
            tunnel: ["rms" "pk"] -> w106
            frame "rms", Default {
            }
            frame "pk" {
            }
          }
          n86 = Less Or Equal?(x=w76, y=T6."W") -> (x <= y?=w85:bool)
          n87 = Equal?(x=w76, y=T6."V") -> (x = y?=w75:bool)
          n88 = Greater Or Equal?(x=w76, y=T6."dBV") -> (x >= y?=w77:bool)
          n89 = Or(x=w75, y=w77) -> (x .or. y?=w74:bool)
          n90 = case shown="\"W\"..\"dBW\"" w76 {
            tunnel: w105 -> [w139 _]
            tunnel: [w138 ""] -> w91
            frame "W".."dBW" {
              n91 = Number To Decimal String(number=w139) -> (decimal integer string=w140:string)  [unwired: 1 out]
              n92 = Concatenate Strings("(" ("Substring"), w140, " ohms)" ("Substring")) -> (w138:string)
            }
            frame Default {
            }
          }
          n93 = case shown="False" w80 {
            tunnel: [w121 w126] -> w79
            tunnel: w74 -> [w122 w125]
            frame False {
              n94 = Select(t="", s=w122, f="^2") -> (s? t:f=w121:string)
            }
            frame True {
              n95 = Select(t="/rtHz", s=w125, f="^2/Hz") -> (s? t:f=w126:string)
            }
          }
          n96 = Select(t=enum16{"linear", "dB"}."linear" ("linear/dB"), s=w85, f=enum16{"linear", "dB"}."dB" ("linear/dB")) -> (s? t:f=w81:enum16{"linear", "dB"})
          n97 = Select(t=T5."Amplitude [Magnitude]" ("spectrum type"), s=w74, f=T5."Power [Magnitude^2]" ("spectrum type")) -> (s? t:f=w86:T5)
          n98 = call "Space Constant.vi"() -> ("String"=w104:string)
          n99 = Bundle By Name(cluster=w99, "spectrum type"=w86, "linear/dB"=w81) -> (w98:T1)
          n100 = Bundle By Name(cluster=w95, "spectrum"=w100) -> (w120:T4)
          n101 = Concatenate Strings(w72, w104, w106, w79, w91) -> (w102:string)
          n102 = Bundle(w103, w102) -> (w101:cluster{string, string})  [unwired: 1 in]
        }
      }
    }
    frame Error {
    }
  }
  "unit converted spectrum" <- w9
  "spectral info out" <- w3
  "error out" <- w1
  "units and label" <- w5
